vi "ricalcolo grandezze.vi"(7 "^2?":bool, 8 "grandezza nom":dbl, 9 "V":dbl, 10 "Vn":dbl, 11 "grandezza":dbl) -> (1 "grandezza ric. /nom.":dbl, 2 "grandezza ric.":dbl)   [LabVIEW 2019]
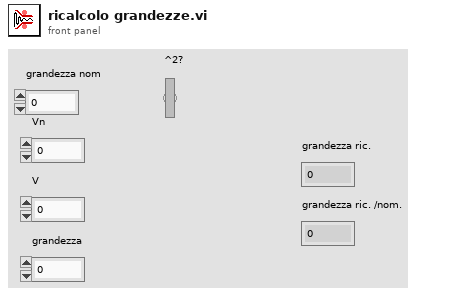
[diagram p1: front panel]
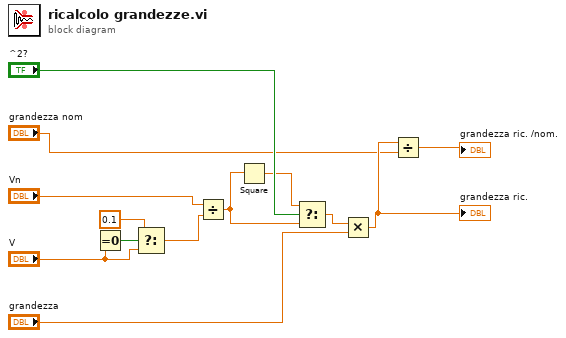
[diagram p0: block diagram]
diagram:
  n1 = Equal To 0?(x="V") -> (x = 0?=w8:bool)
  n2 = Select(t=0.1, s=w8, f="V") -> (s? t:f=w5:dbl)
  n3 = Divide(x="Vn", y=w5) -> (x/y=w9:dbl)
  n4 = Square(x=w9) -> (x^2=w10:dbl)
  n5 = Select(t=w10, s="^2?", f=w9) -> (s? t:f=w12:dbl)
  n6 = Multiply(x=w12, y="grandezza") -> (x*y=w4:dbl)
  "grandezza ric." <- w4
  n7 = Divide(x=w4, y="grandezza nom") -> (x/y=→"grandezza ric. /nom.":dbl)
